vi "main code -click this.vi"() -> ()   [LabVIEW 2014]
uses:
  globalvariables.vi
panel:
  in  "stop":bool
  in  "Cluster":cluster{"OK Button":bool, "OK Button 2":bool}
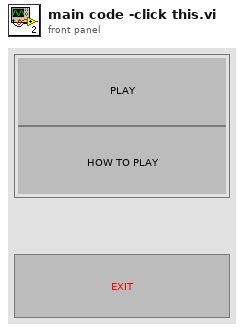
[diagram p1: front panel]
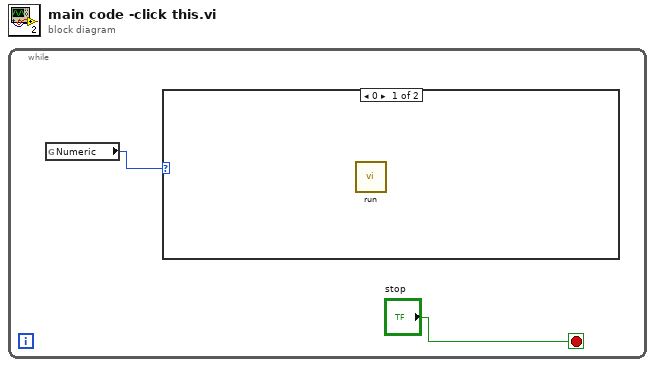
[diagram p0: block diagram]
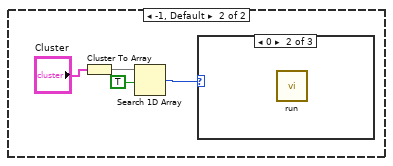
[diagram p2: hidden frame]
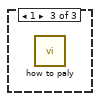
[diagram p4: hidden frame]
diagram:
  n1 = while {
    stop <- "stop" stop-if-true
    n2 = global read "globalvariables.vi" "Numeric"() -> (w1:i8)
    n3 = case shown="0" w1 {
      frame 0 {
        n4 = call "run.vi"() -> ()  [unwired: 12 in]
      }
      frame -1, Default {
        n5 = Cluster To Array(cluster="Cluster") -> (array=w5:bool[])
        n6 = Search 1D Array(1D array=w5, element=TRUE) -> (index of element=w3:i32)  [unwired: 1 in]
        n7 = case shown="0" w3 {
          frame -1, Default {
          }
          frame 0 {
            n8 = call "run.vi"() -> ()  [unwired: 12 in]
          }
          frame 1 {
            n9 = call "how to paly.vi"() -> ()  [unwired: 12 in]
          }
        }
      }
    }
  }
